vi "启动.vi"   [LabVIEW 2016]
uses:
  <vilib>/addons/WireFlow/_WF_ProgressBar.llb/MessageTextType.ctl
  <vilib>/addons/WireFlow/_WF_ProgressBar.llb/WindowBehavior.ctl
  <vilib>/Utility/miscctls.llb/LVRectTypeDef.ctl
  <vilib>/addons/WireFlow/_WF_ProgressBar.llb/ProgressBar_WireFlow.lvclass
types:
  T1 = typedef "ProgressBar_WireFlow.lvclass/WindowBehavior.ctl" = enum16{"No change", "Modal", "Floating"}
  T2 = typedef "ProgressBar_WireFlow.lvclass/MessageTextType.ctl" = enum16{"Title", "General", "Current item"}
  T3 = enum32{"Invalid", "Standard", "Closed", "Hidden", "Minimized", "Maximized"}
  T4 = typedef "LVRectTypeDef.ctl" = cluster{"Left":i16, "Top":i16, "Right":i16, "Bottom":i16}
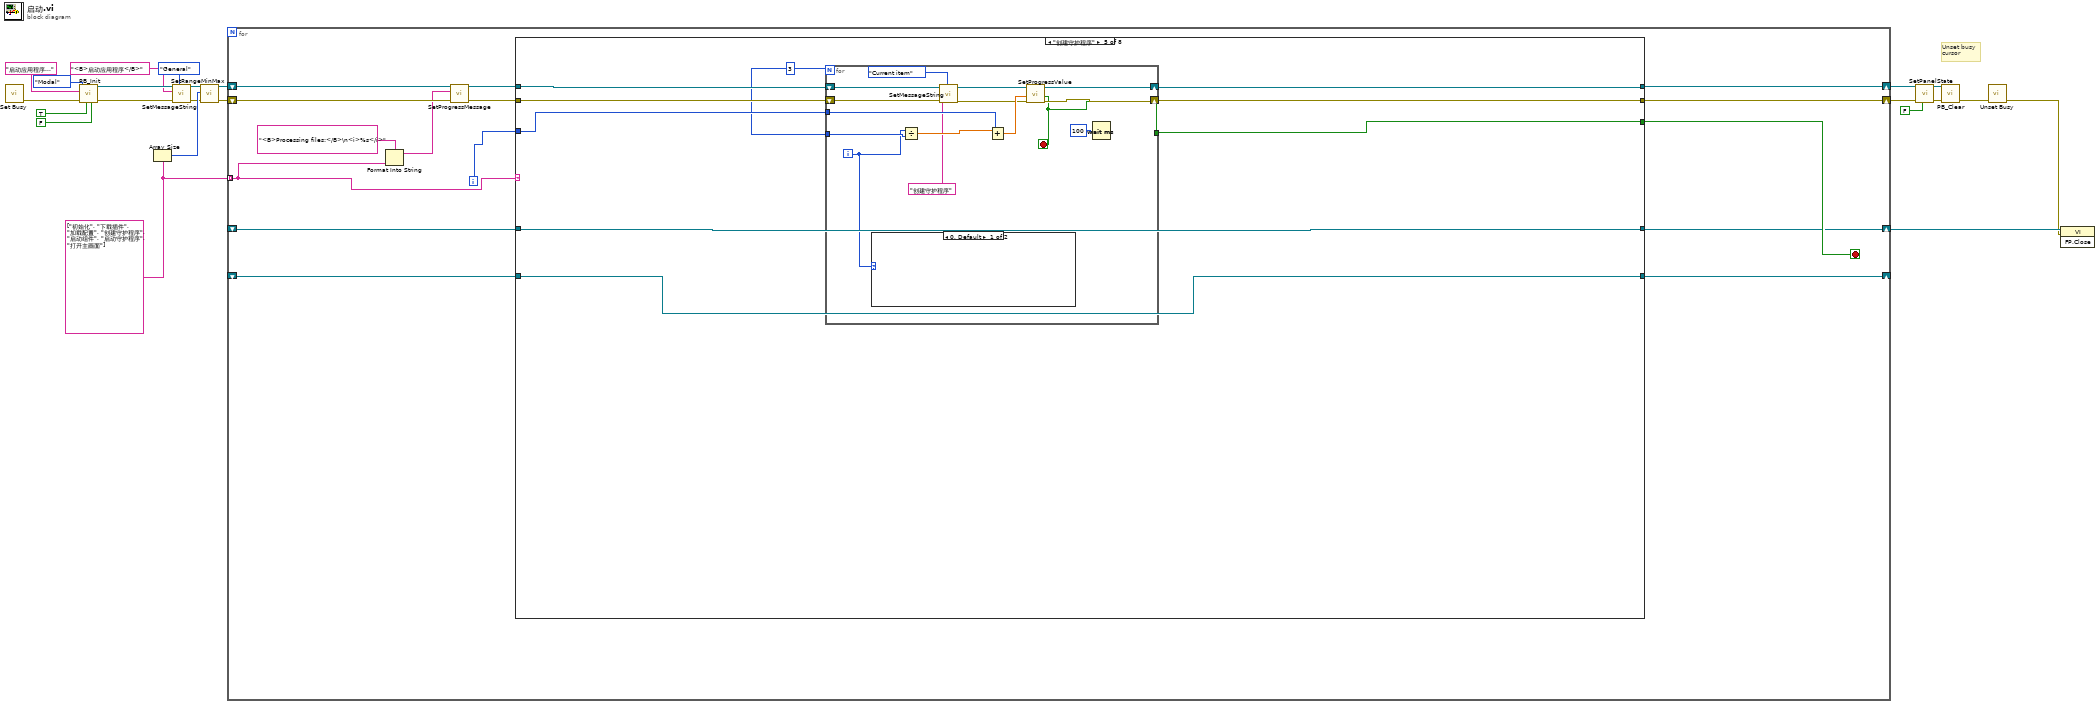
[diagram p0: block diagram]
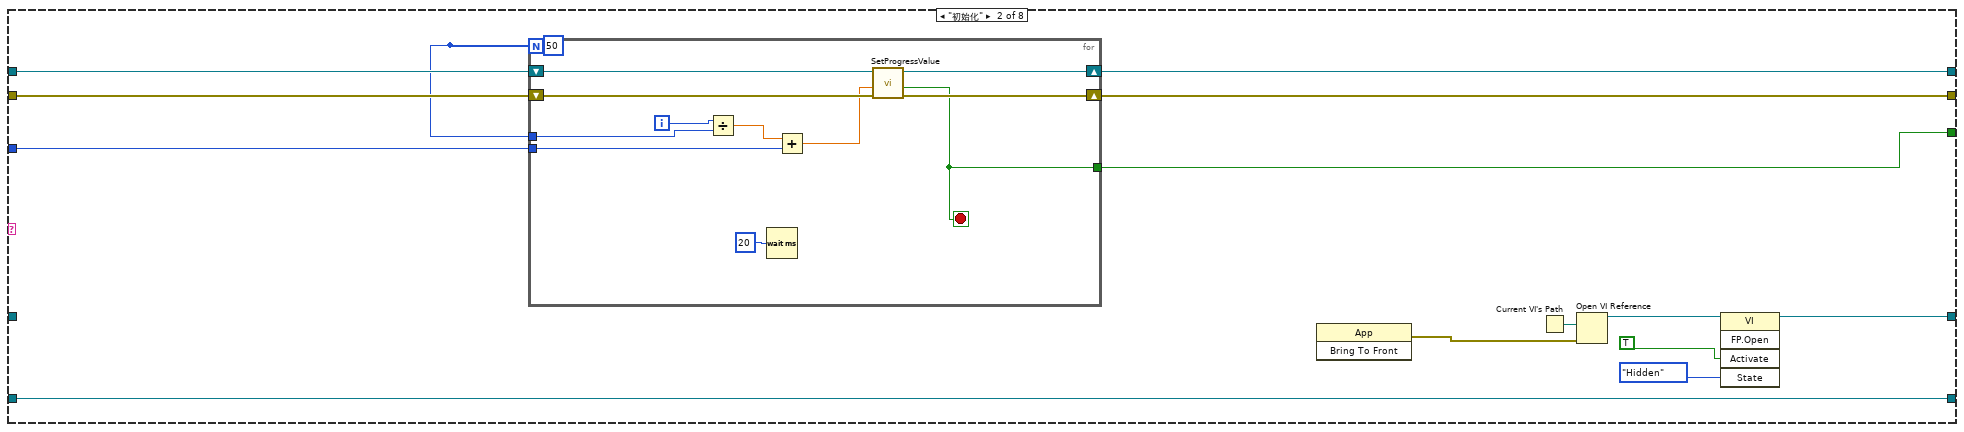
[diagram p3: hidden frame]
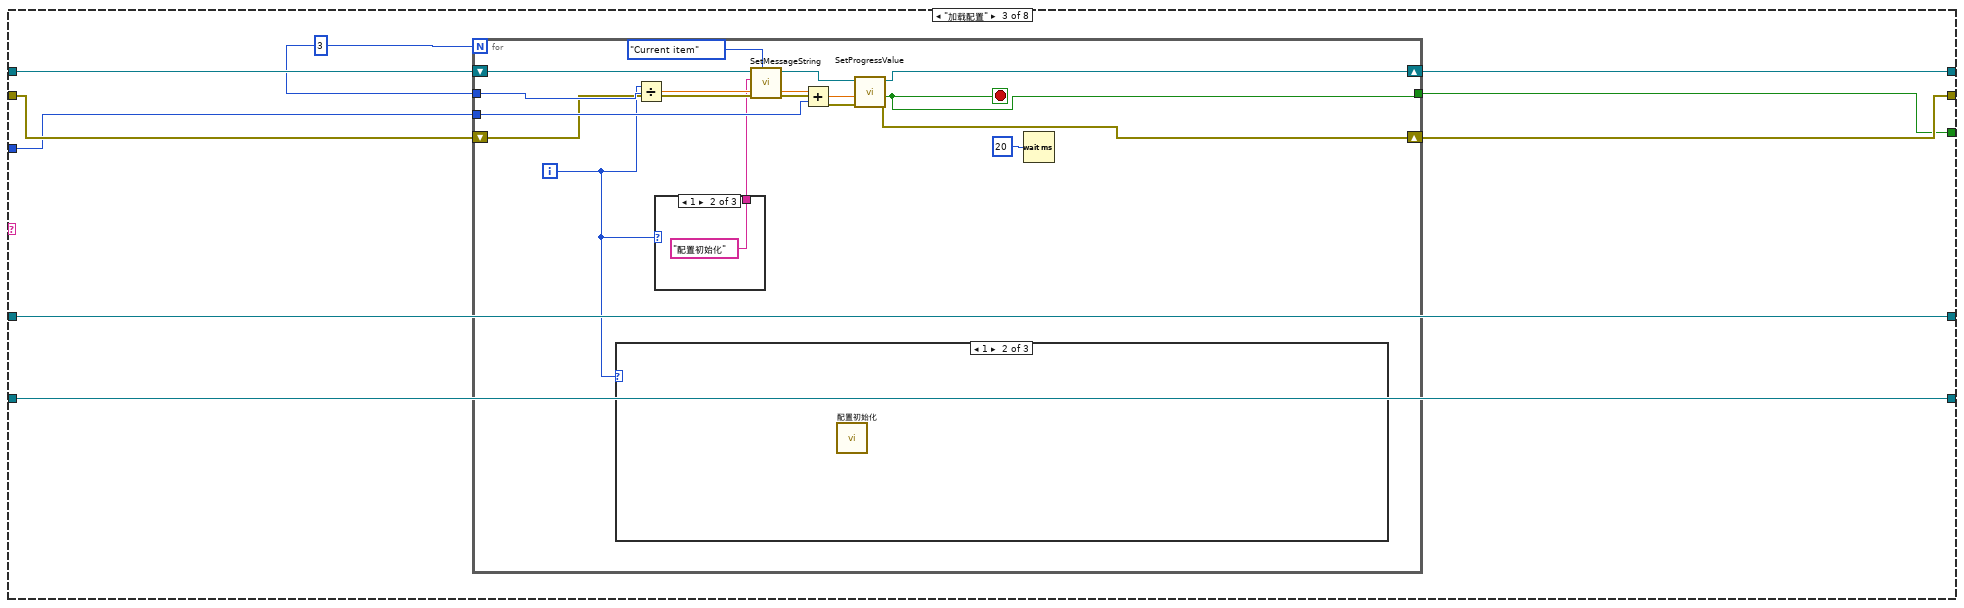
[diagram p4: hidden frame]
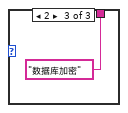
[diagram p6: hidden frame]
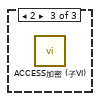
[diagram p8: hidden frame]
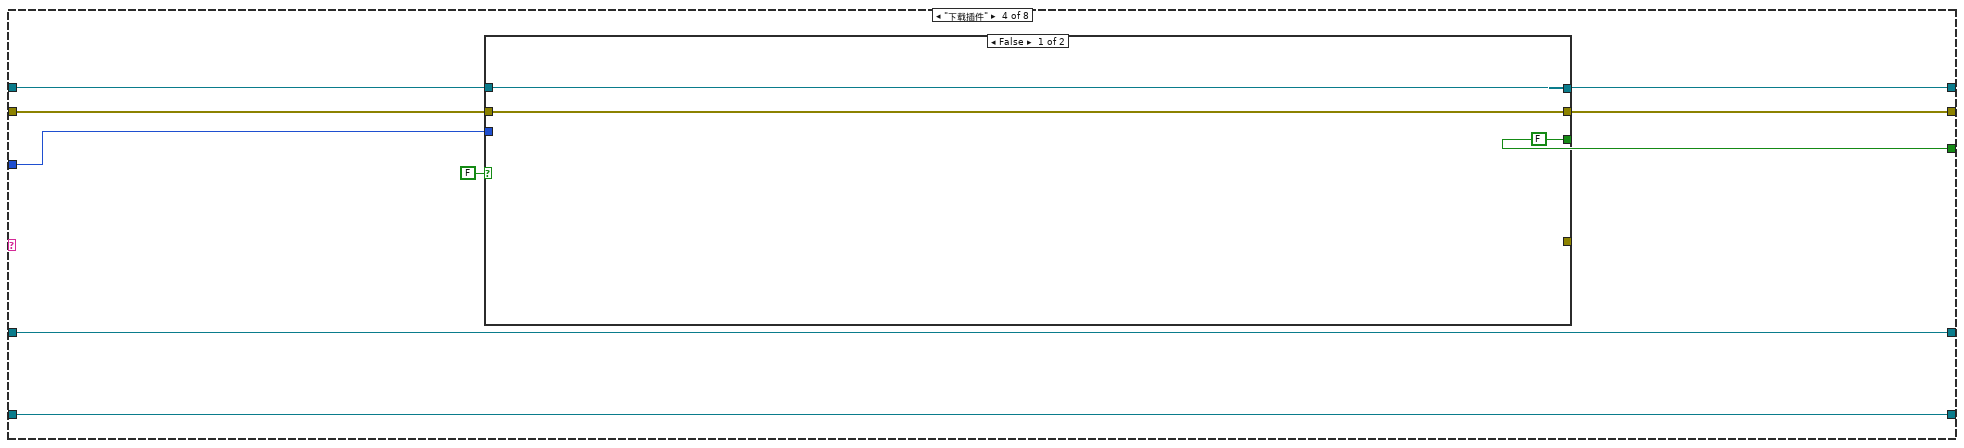
[diagram p9: hidden frame]
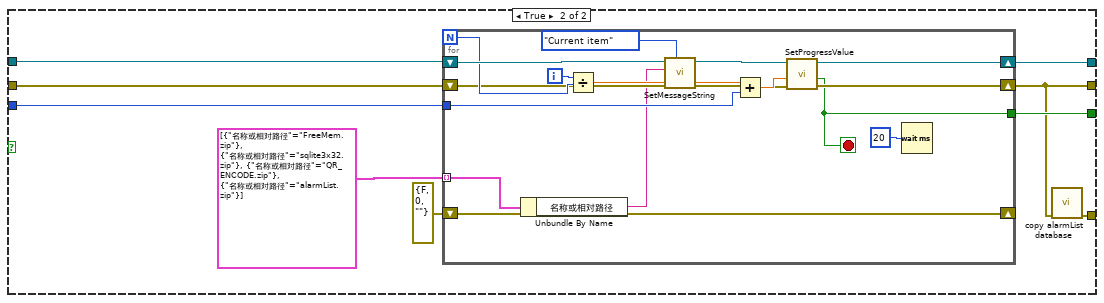
[diagram p10: hidden frame]
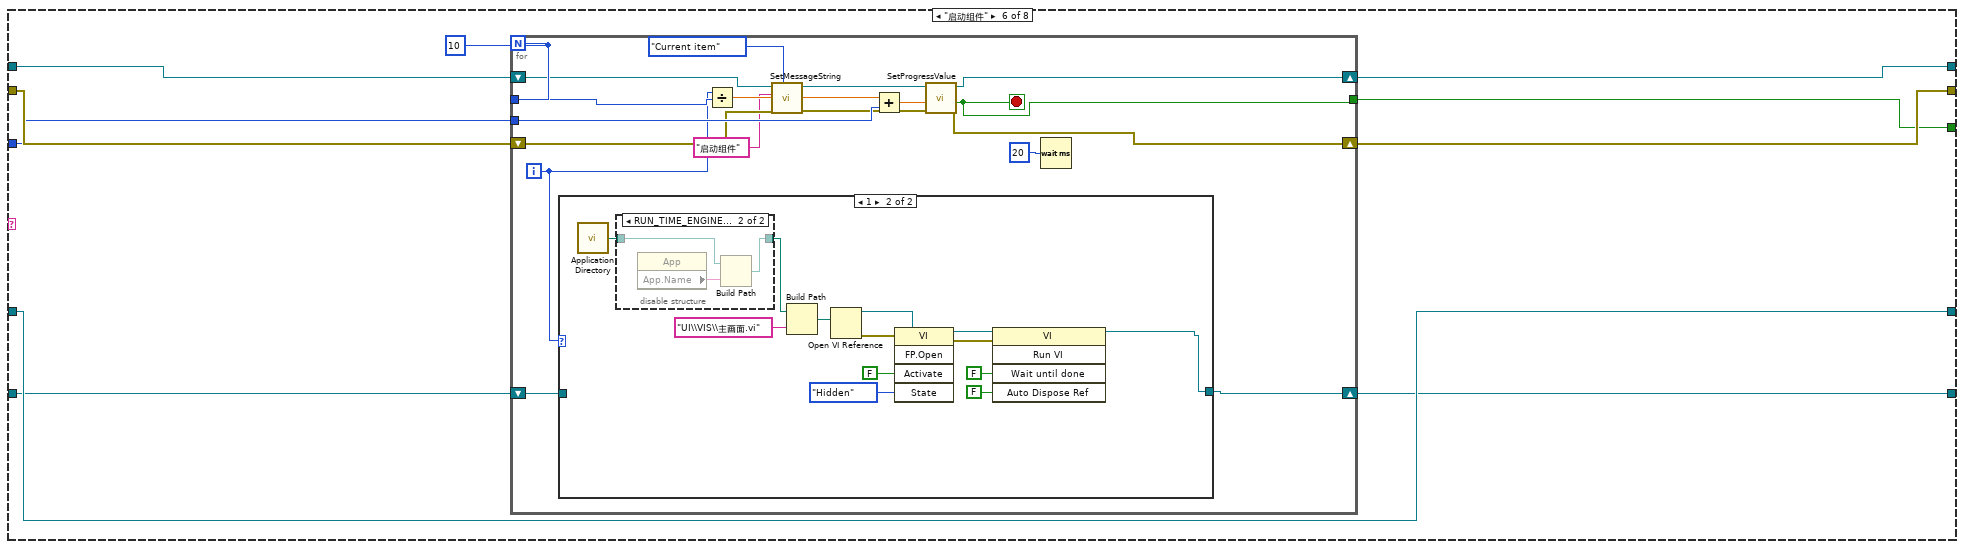
[diagram p12: hidden frame]
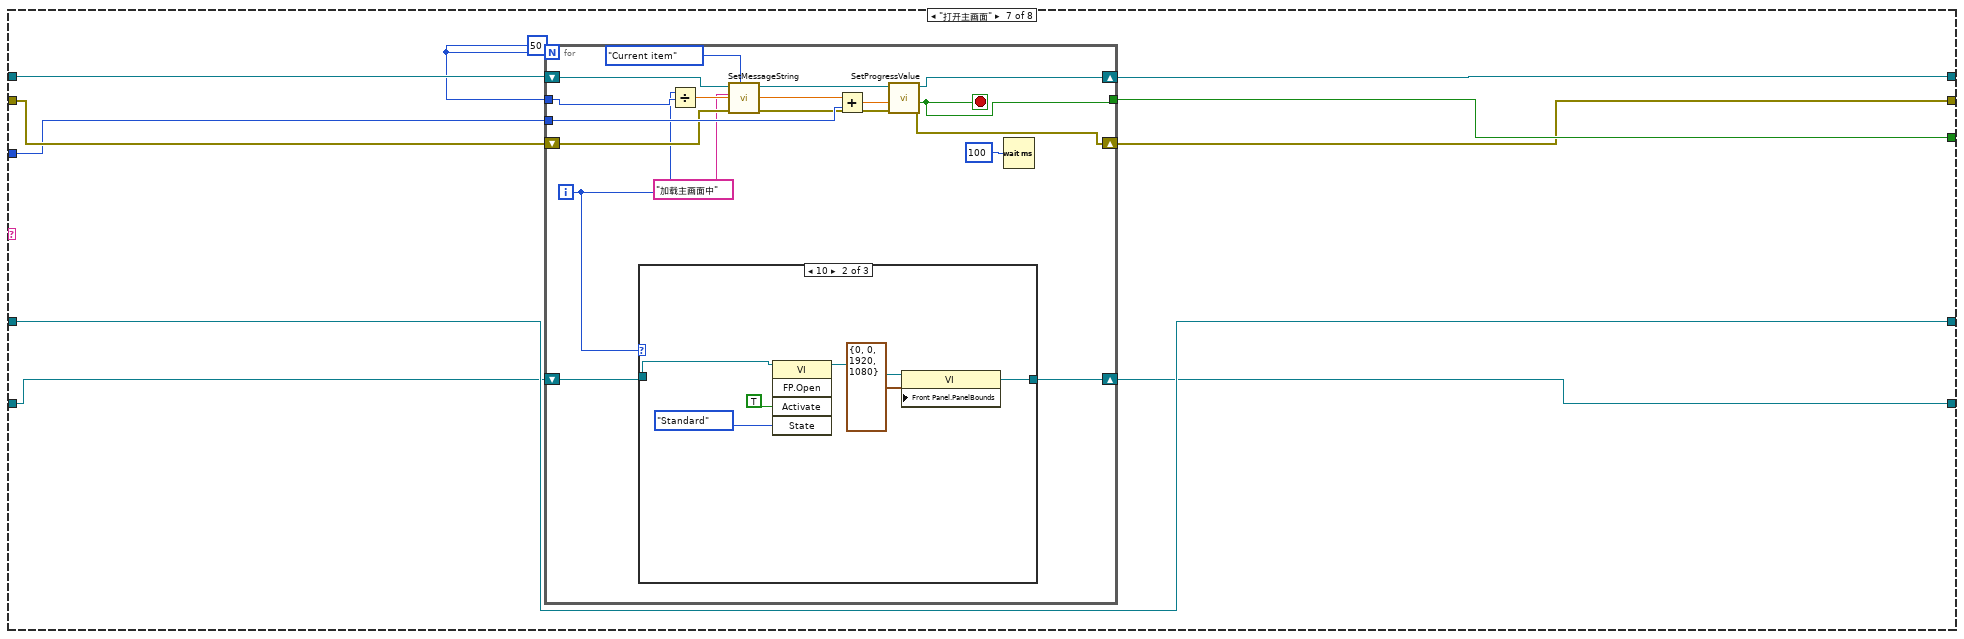
[diagram p15: hidden frame]
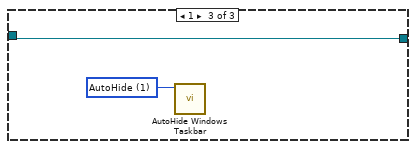
[diagram p17: hidden frame]
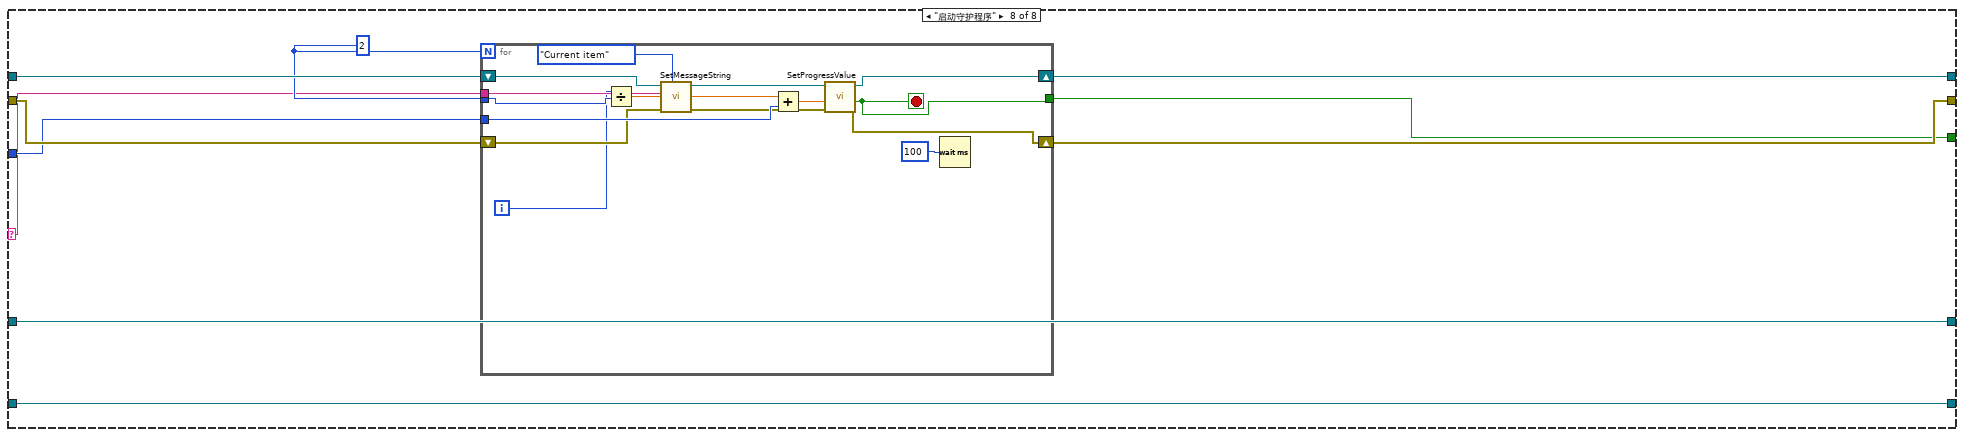
[diagram p18: hidden frame]
diagram:
  w18 = string[] ["初始化", "下载插件", "加载配置", "创建守护程序", "启动组件", "启动守护程序", "打开主画面"]
  # "Unset busy cursor"
  n1 = call <vilib>:"Set Busy.vi"() -> ("error out"=w8:errorcluster)  [unwired: 10 in, 1 out]
  n2 = call <vilib>:"PB_Init.vi"("Cancel button active? (False)"=FALSE ("Cancel active?"), "Open (TRUE)"=TRUE, "error in (no error)"=w8, "Window behavior (No change)"=WindowBehavior."Modal", "title (\"Progress\")"="启动应用程序..." ("title (\"Progress\")")) -> ("error out"=w12:errorcluster, "WF-ProgressBar out"=w14:refnum<class "ProgressBar_WireFlow.lvclass">)  [unwired: 5 in]
  n3 = Array Size(array=w18) -> (size(s)=w19:i32)
  n4 = call-dynamic "SetMessageString.vi"("message field"=MessageTextType."General", "error in (no error)"=w12, "Message"="<B>启动应用程序</B>", "WF-ProgressBar in"=w14) -> ("error out"=w11:errorcluster, "WF-ProgressBar out"=w13:refnum<class "ProgressBar_WireFlow.lvclass">)  [unwired: 6 in]
  n5 = call-dynamic "SetRangeMinMax.vi"("error in (no error)"=w11, "Max (1)"=w19, "WF-ProgressBar in"=w13) -> ("error out"=w4:errorcluster, "WF-ProgressBar out"=w5:refnum<class "ProgressBar_WireFlow.lvclass">)  [unwired: 7 in]
  n6 = for {
    shift-right: [w36] -> w20
    shift-left: w5 -> [w38]
    shift-right: [w30] -> w21
    shift-left: w4 -> [w35]
    tunnel: w18 -> [w28] mode=indexing
    shift-right: [w27] -> w3
    shift-left: _ -> [w26]
    shift-right: [w25] -> _
    shift-left: _ -> [w24]
    i -> [w31]
    stop <- w29 stop-if-true
    n7 = Format Into String(format string="<B>Processing files:</B>\n<i>%s</i>", w28) -> (resulting string=w32:string)  [unwired: 2 in, 1 out]
    n8 = call-dynamic "SetProgressMessage.vi"("error in (no error)"=w35, "Message"=w32, "WF-ProgressBar in"=w38) -> ("error out"=w34:errorcluster, "WF-ProgressBar out"=w37:refnum<class "ProgressBar_WireFlow.lvclass">)  [unwired: 6 in, 1 out]
    n9 = case shown="\"创建守护程序\"" w28 {
      selector: w28 -> [_ _ _ _ _ _ _ w237]
      tunnel: w37 -> [w42 w56 w76 w102 w140 w165 w210 w246]
      tunnel: [w42 w55 w75 w101 w139 w164 w209 w245] -> w36
      tunnel: w34 -> [w41 w54 w74 w100 w138 w163 w208 w244]
      tunnel: w31 -> [_ w53 w73 w99 w137 w162 w207 w243]
      tunnel: [w41 w51 w71 w98 w135 w160 w203 w241] -> w30
      tunnel: [_ w50 w70 w97 w134 w159 w205 w240] -> w29
      tunnel: [w40 w45 w69 w96 w133 w158 w204 w238] -> w27
      tunnel: w26 -> [w40 _ w69 w96 w133 w158 w204 w238]
      tunnel: [w39 w44 w68 w95 w132 w157 w201 w239] -> w25
      tunnel: w24 -> [w39 w44 w68 w95 w132 w156 w202 w239]
      frame Default {
      }
      frame "初始化" {
        w52 = 50
        n10 = for {
          N: w52 -> [_]
          tunnel: w53 -> [w62]
          shift-right: [w66] -> w55
          shift-left: w56 -> [w67]
          shift-right: [w58] -> w51
          shift-left: w54 -> [w65]
          tunnel: w52 -> [w59]
          tunnel: [w57] -> w50
          i -> [w64]
          stop <- w57 stop-if-true
          n11 = Divide(x=w64, y=w59) -> (x/y=w63:dbl)
          n12 = Wait (ms)(milliseconds to wait=u32 20) -> ()  [unwired: 1 out]
          n13 = Add(x=w63, y=w62) -> (x+y=w61:dbl)
          n14 = call-dynamic "SetProgressValue.vi"("error in (no error)"=w65, "Value"=w61, "WF-ProgressBar in"=w67) -> ("error out"=w58:errorcluster, "cancelled?"=w57:bool, "WF-ProgressBar out"=w66:refnum<class "ProgressBar_WireFlow.lvclass">)  [unwired: 6 in]
        }
        n15 = invoke class="App" method="Bring To Front"() -> (error out=w43:errorcluster)  [unwired: 3 in, 2 out]
        n16 = Current VI's Path() -> (path=w47:path)
        n17 = Open VI Reference(vi path=w47, error in (no error)=w43) -> (vi reference=w46:refnum<vi>)  [unwired: 4 in, 1 out]
        n18 = invoke class="VI" method="FP.Open"(reference=w46, "Activate"=TRUE ("激活？"), "State"=T3."Hidden" ("状态")) -> (reference out=w45:refnum<vi>)  [unwired: 2 in, 4 out]
      }
      frame "加载配置" {
        w72 = 3
        n19 = for {
          N: w72 -> [_]
          tunnel: w73 -> [w88]
          shift-right: [w90] -> w75
          shift-left: w76 -> [w91]
          shift-right: [w84] -> w71
          shift-left: w74 -> [w81]
          tunnel: w72 -> [w85]
          tunnel: [w83] -> w70
          i -> [w78]
          stop <- w83 stop-if-true
          n20 = case shown="1" w78 {
            frame 0, Default {
            }
            frame 1 {
              n21 = call "配置初始化.vi"() -> ()  [unwired: 11 in, 1 out]
            }
            frame 2 {
              n22 = call "ACCESS加密 (子VI).vi"() -> ()  [unwired: 11 in, 1 out]
            }
          }
          n23 = Divide(x=w78, y=w85) -> (x/y=w89:dbl)
          n24 = case shown="1" w78 {
            tunnel: [_ "配置初始化" "数据库加密"] -> w77
            frame 0, Default {
            }
            frame 1 {
            }
            frame 2 {
            }
          }
          n25 = call-dynamic "SetMessageString.vi"("message field"=MessageTextType."Current item", "error in (no error)"=w81, "Message"=w77, "WF-ProgressBar in"=w91) -> ("error out"=w80:errorcluster, "WF-ProgressBar out"=w82:refnum<class "ProgressBar_WireFlow.lvclass">)  [unwired: 6 in]
          n26 = Add(x=w89, y=w88) -> (x+y=w87:dbl)
          n27 = call-dynamic "SetProgressValue.vi"("error in (no error)"=w80, "Value"=w87, "WF-ProgressBar in"=w82) -> ("error out"=w84:errorcluster, "cancelled?"=w83:bool, "WF-ProgressBar out"=w90:refnum<class "ProgressBar_WireFlow.lvclass">)  [unwired: 6 in]
          n28 = Wait (ms)(milliseconds to wait=u32 20) -> ()  [unwired: 1 out]
        }
      }
      frame "下载插件" {
        n29 = case shown="False" FALSE {
          tunnel: w102 -> [w105 w114]
          tunnel: [w105 w113] -> w101
          tunnel: w100 -> [w104 w112]
          tunnel: w99 -> [_ w111]
          tunnel: [w104 w108] -> w98
          tunnel: [FALSE ("cancelled?") w110] -> w97
          tunnel: [_ w107] -> _
          frame False {
          }
          frame True {
            n30 = for {
              N -> [w121]
              tunnel: w111 -> [w127]
              shift-right: [w130] -> w113
              shift-left: w114 -> [w131]
              shift-right: [w124] -> w108
              shift-left: w112 -> [w119]
              tunnel: [w123] -> w110
              tunnel: cluster{"名称或相对路径":string}[] [{"名称或相对路径"="FreeMem.zip"}, {"名称或相对路径"="sqlite3x32.zip"}, {"名称或相对路径"="QR_ENCODE.zip"}, {"名称或相对路径"="alarmList.zip"}] -> [w122] mode=indexing
              shift-right: [w115] -> _
              shift-left: errorcluster {"status"=FALSE, "code"=0, "source"=""} ("error out") -> [w115]
              i -> [w129]
              stop <- w123 stop-if-true
              n31 = Unbundle By Name(w122) -> ("名称或相对路径"=w116:string)
              n32 = Divide(x=w129, y=w121) -> (x/y=w128:dbl)
              n33 = call-dynamic "SetMessageString.vi"("message field"=MessageTextType."Current item", "error in (no error)"=w119, "Message"=w116, "WF-ProgressBar in"=w131) -> ("error out"=w118:errorcluster, "WF-ProgressBar out"=w120:refnum<class "ProgressBar_WireFlow.lvclass">)  [unwired: 6 in]
              n34 = Add(x=w128, y=w127) -> (x+y=w126:dbl)
              n35 = call-dynamic "SetProgressValue.vi"("error in (no error)"=w118, "Value"=w126, "WF-ProgressBar in"=w120) -> ("error out"=w124:errorcluster, "cancelled?"=w123:bool, "WF-ProgressBar out"=w130:refnum<class "ProgressBar_WireFlow.lvclass">)  [unwired: 6 in]
              n36 = Wait (ms)(milliseconds to wait=u32 20) -> ()  [unwired: 1 out]
            }
            n37 = call "copy alarmList database.vi"("error in (no error)"=w108) -> ("error out"=w107:errorcluster)  [unwired: 10 in]
          }
        }
      }
      frame "创建守护程序" {
        w136 = 3
        n38 = for {
          N: w136 -> [_]
          tunnel: w137 -> [w152]
          shift-right: [w154] -> w139
          shift-left: w140 -> [w155]
          shift-right: [w148] -> w135
          shift-left: w138 -> [w145]
          tunnel: w136 -> [w149]
          tunnel: [w147] -> w134
          i -> [w143]
          stop <- w147 stop-if-true
          n39 = case shown="0, Default" w143 {
            frame 0, Default {
            }
            frame 1 {
            }
          }
          n40 = Divide(x=w143, y=w149) -> (x/y=w153:dbl)
          n41 = call-dynamic "SetMessageString.vi"("message field"=MessageTextType."Current item", "error in (no error)"=w145, "Message"="创建守护程序", "WF-ProgressBar in"=w155) -> ("error out"=w144:errorcluster, "WF-ProgressBar out"=w146:refnum<class "ProgressBar_WireFlow.lvclass">)  [unwired: 6 in]
          n42 = Add(x=w153, y=w152) -> (x+y=w151:dbl)
          n43 = call-dynamic "SetProgressValue.vi"("error in (no error)"=w144, "Value"=w151, "WF-ProgressBar in"=w146) -> ("error out"=w148:errorcluster, "cancelled?"=w147:bool, "WF-ProgressBar out"=w154:refnum<class "ProgressBar_WireFlow.lvclass">)  [unwired: 6 in]
          n44 = Wait (ms)(milliseconds to wait=u32 100) -> ()  [unwired: 1 out]
        }
      }
      frame "启动组件" {
        w161 = 10
        n45 = for {
          N: w161 -> [_]
          tunnel: w162 -> [w179]
          shift-right: [w181] -> w164
          shift-left: w165 -> [w182]
          shift-right: [w175] -> w160
          shift-left: w163 -> [w169]
          tunnel: w161 -> [w176]
          tunnel: [w174] -> w159
          shift-right: [w173] -> w157
          shift-left: w156 -> [w171]
          i -> [w172]
          stop <- w174 stop-if-true
          n46 = case shown="1" w172 {
            tunnel: [w183 w191] -> w173
            tunnel: w171 -> [w183 _]
            frame Default {
            }
            frame 1 {
              n47 = call <vilib>:"Application Directory.vi"() -> ("Application Directory"=w193:path)
              n48 = disable-structure shown="RUN_TIME_ENGINE==True" {
                disable-tunnel: w193 -> [w197 w200]
                disable-tunnel: [w197 w198] -> w192
                frame condition #0 (active) {
                }
                frame condition #1 {
                  n49 = property class="App"() -> ("App.Name"=w199:string)  [unwired: 2 in, 2 out]
                  n50 = Build Path(base path=w200, name or relative path=w199) -> (appended path=w198:path)
                }
              }
              n51 = Build Path(base path=w192, name or relative path="UI\\VIS\\主画面.vi" ("名称或相对路径")) -> (appended path=w184:path)
              n52 = Open VI Reference(vi path=w184) -> (vi reference=w190:refnum<vi>, error out=w188:errorcluster)  [unwired: 5 in]
              n53 = invoke class="VI" method="FP.Open"(reference=w190, error in=w188, "Activate"=FALSE ("激活？"), "State"=T3."Hidden" ("状态")) -> (reference out=w189:refnum<vi>, error out=w187:errorcluster)  [unwired: 1 in, 3 out]
              n54 = invoke class="VI" method="Run VI"(reference=w189, error in=w187, "Wait until done"=FALSE ("结束前等待"), "Auto Dispose Ref"=FALSE ("自动销毁引用")) -> (reference out=w191:refnum<vi>)  [unwired: 1 in, 4 out]
            }
          }
          n55 = Divide(x=w172, y=w176) -> (x/y=w180:dbl)
          n56 = call-dynamic "SetMessageString.vi"("message field"=MessageTextType."Current item", "error in (no error)"=w169, "Message"="启动组件", "WF-ProgressBar in"=w182) -> ("error out"=w168:errorcluster, "WF-ProgressBar out"=w170:refnum<class "ProgressBar_WireFlow.lvclass">)  [unwired: 6 in]
          n57 = Add(x=w180, y=w179) -> (x+y=w178:dbl)
          n58 = call-dynamic "SetProgressValue.vi"("error in (no error)"=w168, "Value"=w178, "WF-ProgressBar in"=w170) -> ("error out"=w175:errorcluster, "cancelled?"=w174:bool, "WF-ProgressBar out"=w181:refnum<class "ProgressBar_WireFlow.lvclass">)  [unwired: 6 in]
          n59 = Wait (ms)(milliseconds to wait=u32 20) -> ()  [unwired: 1 out]
        }
      }
      frame "打开主画面" {
        w206 = 50
        n60 = for {
          N: w206 -> [_]
          tunnel: w207 -> [w224]
          shift-right: [w226] -> w209
          shift-left: w210 -> [w227]
          shift-right: [w220] -> w203
          shift-left: w208 -> [w216]
          tunnel: w206 -> [w221]
          tunnel: [w219] -> w205
          shift-right: [w211] -> w201
          shift-left: w202 -> [w212]
          i -> [w213]
          stop <- w219 stop-if-true
          n61 = case shown="10" w213 {
            tunnel: w212 -> [w228 w232 w236]
            tunnel: [w228 w230 w236] -> w211
            frame 0, Default {
            }
            frame 10 {
              n62 = invoke class="VI" method="FP.Open"(reference=w232, "Activate"=TRUE ("激活？"), "State"=T3."Standard" ("状态")) -> (reference out=w231:refnum<vi>)  [unwired: 2 in, 4 out]
              n63 = property class="VI"(reference=w231, "Front Panel.PanelBounds"=T4 {"Left"=0, "Top"=0, "Right"=1920, "Bottom"=1080} ("前面板窗口:窗口边界")) -> (reference out=w230:refnum<vi>)  [unwired: 1 in, 1 out]
            }
            frame 1 {
              w235 = u8 1 items=["AutoHide"=1, "AlwaysOnTop"=2] ("Operation")
              n64 = call "AutoHide Windows Taskbar.vi"("Operation"=w235) -> ()  [unwired: 6 in, 1 out]
            }
          }
          n65 = Divide(x=w213, y=w221) -> (x/y=w225:dbl)
          n66 = call-dynamic "SetMessageString.vi"("message field"=MessageTextType."Current item", "error in (no error)"=w216, "Message"="加载主画面中", "WF-ProgressBar in"=w227) -> ("error out"=w215:errorcluster, "WF-ProgressBar out"=w218:refnum<class "ProgressBar_WireFlow.lvclass">)  [unwired: 6 in]
          n67 = Add(x=w225, y=w224) -> (x+y=w223:dbl)
          n68 = call-dynamic "SetProgressValue.vi"("error in (no error)"=w215, "Value"=w223, "WF-ProgressBar in"=w218) -> ("error out"=w220:errorcluster, "cancelled?"=w219:bool, "WF-ProgressBar out"=w226:refnum<class "ProgressBar_WireFlow.lvclass">)  [unwired: 6 in]
          n69 = Wait (ms)(milliseconds to wait=u32 100) -> ()  [unwired: 1 out]
        }
      }
      frame "启动守护程序" {
        w242 = 2
        n70 = for {
          N: w242 -> [_]
          tunnel: w243 -> [w258]
          shift-right: [w260] -> w245
          shift-left: w246 -> [w261]
          shift-right: [w254] -> w241
          shift-left: w244 -> [w251]
          tunnel: w242 -> [w255]
          tunnel: [w253] -> w240
          tunnel: w237 -> [w249]
          i -> [w247]
          stop <- w253 stop-if-true
          n71 = Divide(x=w247, y=w255) -> (x/y=w259:dbl)
          n72 = call-dynamic "SetMessageString.vi"("message field"=MessageTextType."Current item", "error in (no error)"=w251, "Message"=w249, "WF-ProgressBar in"=w261) -> ("error out"=w250:errorcluster, "WF-ProgressBar out"=w252:refnum<class "ProgressBar_WireFlow.lvclass">)  [unwired: 6 in]
          n73 = Add(x=w259, y=w258) -> (x+y=w257:dbl)
          n74 = call-dynamic "SetProgressValue.vi"("error in (no error)"=w250, "Value"=w257, "WF-ProgressBar in"=w252) -> ("error out"=w254:errorcluster, "cancelled?"=w253:bool, "WF-ProgressBar out"=w260:refnum<class "ProgressBar_WireFlow.lvclass">)  [unwired: 6 in]
          n75 = Wait (ms)(milliseconds to wait=u32 100) -> ()  [unwired: 1 out]
        }
      }
    }
  }
  n76 = call-dynamic "SetPanelState.vi"("State (T = Open)"=FALSE, "error in (no error)"=w21, "WF-ProgressBar in"=w20) -> ("error out"=w15:errorcluster, "WF-ProgressBar out"=w16:refnum<class "ProgressBar_WireFlow.lvclass">)  [unwired: 7 in]
  n77 = call-dynamic "PB_Clear.vi"("error in (no error)"=w15, "WF-ProgressBar in"=w16) -> ("error out"=w7:errorcluster)  [unwired: 8 in, 1 out]
  n78 = call <vilib>:"Unset Busy.vi"("error in (no error)"=w7) -> ("error out"=w2:errorcluster)  [unwired: 10 in]
  n79 = invoke class="VI" method="FP.Close"(reference=w3, error in=w2) -> ()  [unwired: 1 in, 3 out]
